vi "handle.vi"(9 "枚举":enum16{"write", "read"}(ring), 11 "In Handle":cluster{"Session":u32, "Card number":u32}) -> (3 "Output Handle":cluster{"Session":u32, "Card number":u32})   [LabVIEW 2018]
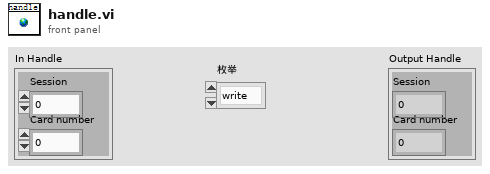
[diagram p1: front panel]
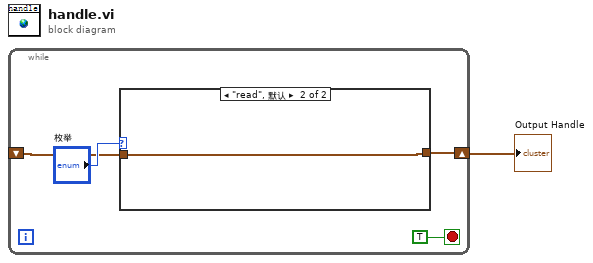
[diagram p0: block diagram]
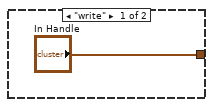
[diagram p2: hidden frame]
diagram:
  n1 = while {
    shift-right: [w3] -> w1
    shift-left: _ -> [w2]
    stop <- TRUE stop-if-true
    n2 = case shown="\"read\", 默认" "枚举" {
      tunnel: ["In Handle" w7] -> w3
      tunnel: w2 -> [_ w7]
      frame "write" {
      }
      frame "read", Default {
      }
    }
  }
  "Output Handle" <- w1
